vi "LVscope.vi"() -> ()   [LabVIEW 2020]
uses:
  <vilib>/Instr/_visa.llb/VISA Configure Serial Port (Instr).vi
panel:
  in  "Rising\n\nFalling":bool
  out "Triggered":bool
  out "run_ind":bool
  in  "Run/Stop":bool=TRUE
  in  "Sample rate":T1(radio)=enum."19.2 kS/s"
  in  "Trigger Voltage":dbl(knob)=2.5 scale=0.0..5.0
  out "Mean (DC)":dbl[unit]
  out "Min":dbl[unit]
  out "Max":dbl[unit]
  out "RMS":dbl[unit]
  in  "tdiv multiplier":enum32{"10us", "ms", "10ms", "100us"}(radio)=enum."ms"
  in  "Time/Div":dbl(knob)=5.0 scale=1.0..10.0
  in  "Volts/Div":sgl(knob)=2.5 caption="Diala" scale=0.1..7.5
  in  "OK Button":bool
  out "Frequency":dbl[unit]
  out "Peak to Peak":dbl[unit]
  out "Waveform Graph":waveform(dbl)(graph)
  in  "exit\nexit":bool
  in  "COM Port":refnum<visa-resource-name>
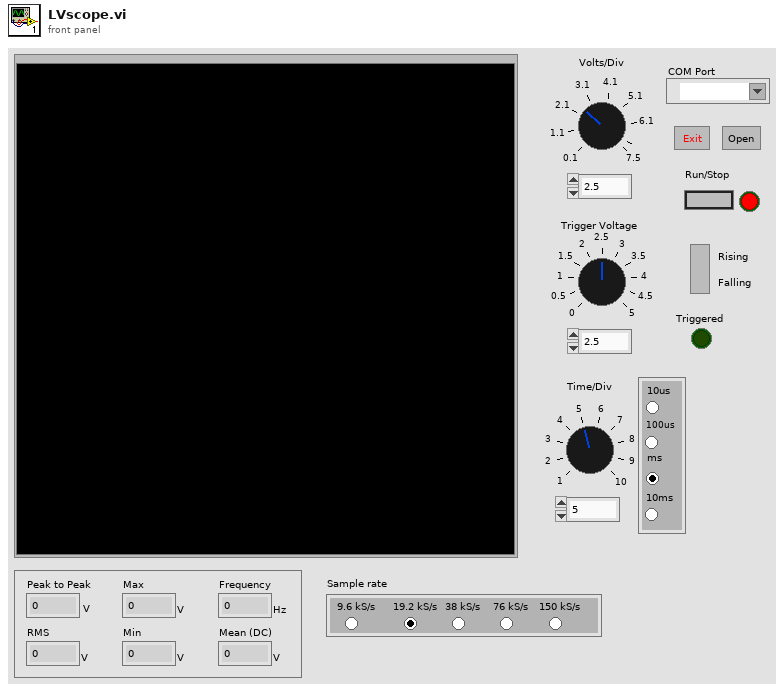
[diagram p1: front panel]
types:
  T1 = enum32{"9.6 kS/s", "19.2 kS/s", "38 kS/s", "76 kS/s", "150 kS/s"}
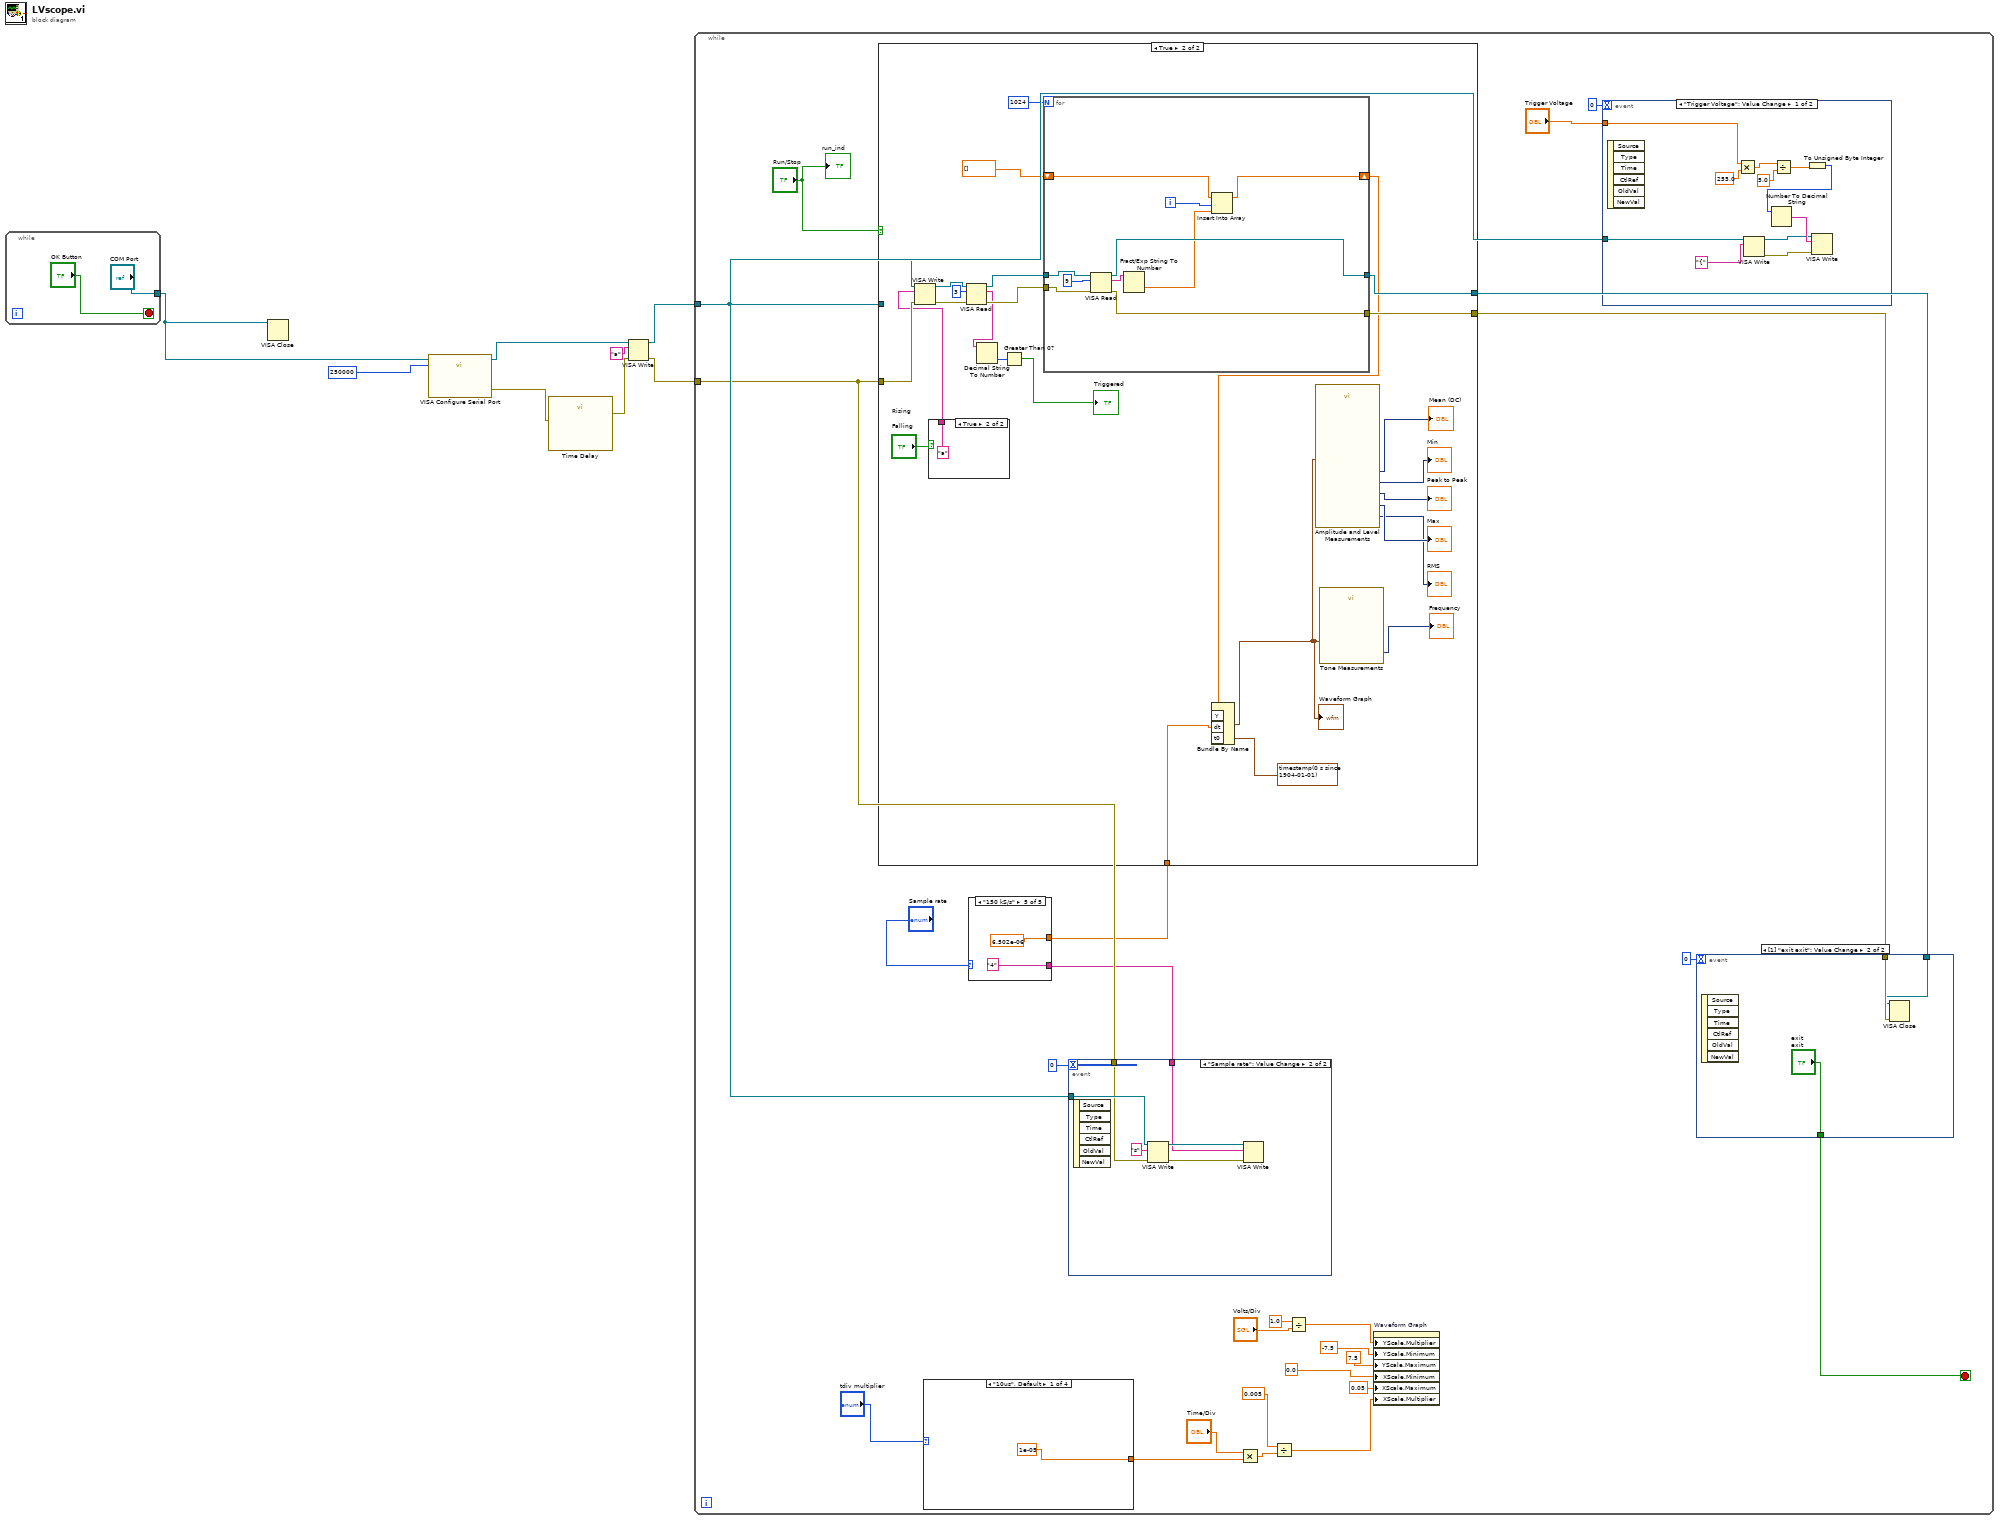
[diagram p0: block diagram]
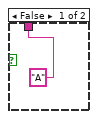
[diagram p3: hidden frame]
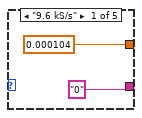
[diagram p4: hidden frame]
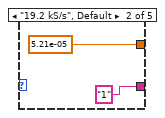
[diagram p5: hidden frame]
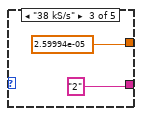
[diagram p6: hidden frame]
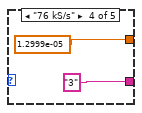
[diagram p7: hidden frame]
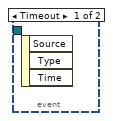
[diagram p8: hidden frame]
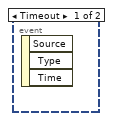
[diagram p9: hidden frame]
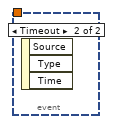
[diagram p10: hidden frame]
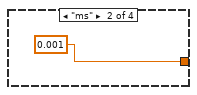
[diagram p11: hidden frame]
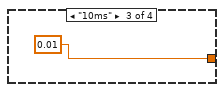
[diagram p12: hidden frame]
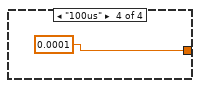
[diagram p13: hidden frame]
diagram:
  n1 = while {
    tunnel: ["COM Port"] -> w2
    stop <- "OK Button" stop-if-true
  }
  n2 = VISA Close(VISA resource name=w2) -> ()  [unwired: 1 in, 1 out]
  n3 = call-poly "VISA Configure Serial Port"("VISA resource name"=w2, "baud rate (9600)"=250000) -> ("VISA resource name out"=w6:refnum<visa-resource-name>, "error out"=w4:errorcluster)  [unwired: 12 in]
  n4 = call "Time Delay"("error in (no error)"=w4) -> ("error out"=w3:errorcluster)  [unwired: 10 in]
  n5 = VISA Write(VISA resource name=w6, write buffer="a", error in (no error)=w3) -> (VISA resource name out=w1:refnum<visa-resource-name>, error out=w5:errorcluster)  [unwired: 1 out]
  n6 = while {
    tunnel: w1 -> [w15]
    tunnel: w5 -> [w14]
    stop <- w21 stop-if-true
    n7 = case shown="\"10us\", Default" "tdiv multiplier" {
      tunnel: [1e-05 0.001 0.01 0.0001] -> w26
      frame "10us", Default {
      }
      frame "ms" {
      }
      frame "10ms" {
      }
      frame "100us" {
      }
    }
    n8 = case shown="\"150 kS/s\"" "Sample rate" {
      tunnel: ["0" "1" "2" "3" "4"] -> w13
      tunnel: [0.000104 5.21e-05 2.59994e-05 1.2999e-05 6.502e-06] -> w11
      frame "9.6 kS/s" {
      }
      frame "19.2 kS/s", Default {
      }
      frame "38 kS/s" {
      }
      frame "76 kS/s" {
      }
      frame "150 kS/s" {
      }
    }
    n9 = case shown="True" "Run/Stop" {
      tunnel: [_ w60] -> w18
      tunnel: [_ w59] -> w17
      tunnel: w15 -> [_ w58]
      tunnel: w14 -> [_ w57]
      tunnel: w11 -> [_ w53]
      frame False {
      }
      frame True {
        n10 = case shown="True" "Rising\n\nFalling" {
          tunnel: ["A" "a"] -> w37
          frame False {
          }
          frame True {
          }
        }
        n11 = VISA Write(VISA resource name=w58, write buffer=w37, error in (no error)=w57) -> (VISA resource name out=w45:refnum<visa-resource-name>, error out=w44:errorcluster)  [unwired: 1 out]
        n12 = VISA Read(VISA resource name=w45, byte count=u32 3, error in (no error)=w44) -> (VISA resource name out=w43:refnum<visa-resource-name>, read buffer=w41:string, error out=w42:errorcluster)  [unwired: 1 out]
        n13 = Decimal String To Number(string=w41) -> (number=w40:i32)  [unwired: 2 in, 1 out]
        n14 = Greater Than 0?(x=w40) -> (x > 0?=→"Triggered":bool)
        n15 = for {
          N: 1024 -> [_]
          tunnel: w43 -> [w74]
          tunnel: [w73] -> w60
          shift-right: [w67] -> w56
          shift-left: dbl[] [] ("array") -> [w68]
          tunnel: w42 -> [w66]
          tunnel: [w65] -> w59
          i -> [w70]
          n16 = VISA Read(VISA resource name=w74, byte count=u32 9, error in (no error)=w66) -> (VISA resource name out=w73:refnum<visa-resource-name>, read buffer=w71:string, error out=w65:errorcluster)  [unwired: 1 out]
          n17 = Fract/Exp String To Number(string=w71) -> (number=w69:dbl)  [unwired: 3 in, 1 out]
          n18 = Insert Into Array(array=w68, index=w70, new element=w69) -> (w67:dbl[])
        }
        n19 = Bundle By Name("Y"=w56, "dt"=w53, "t0"=timestamp(0 s since 1904-01-01)) -> (w54:waveform(dbl))  [unwired: 1 in]
        "Waveform Graph" <- w54
        n20 = call "Amplitude and Level Measurements"("Signals"=w54) -> ("Mean (DC)"=→"Mean (DC)":dynamicdata, "RMS"=→"RMS":dynamicdata, "Negative Peak"=→"Min":dynamicdata, "Positive Peak"=→"Max":dynamicdata, "Peak to Peak"=→"Peak to Peak":dynamicdata)  [unwired: 9 in, 1 out]
        n21 = call "Tone Measurements"("Signals"=w54) -> ("Frequency"=→"Frequency":dynamicdata)  [unwired: 9 in, 1 out]
      }
    }
    n22 = event shown="[1] \"Sample rate\": Value Change" {
      selector: _ -> [_ _]
      dyn-events: _ -> [_ _]
      timeout: 0 -> [_ _]
      tunnel: w15 -> [_ w87]
      tunnel: w14 -> [_ w86]
      tunnel: w13 -> [_ w85]
      event Timeout {
        n23 = event-data() -> ()  [unwired: 1 in, 3 out]
      }
      event "Sample rate": Value Change {
        n24 = event-data() -> ()  [unwired: 1 in, 6 out]
        n25 = VISA Write(VISA resource name=w87, write buffer="s", error in (no error)=w86) -> (VISA resource name out=w89:refnum<visa-resource-name>, error out=w88:errorcluster)  [unwired: 1 out]
        n26 = VISA Write(VISA resource name=w89, write buffer=w85, error in (no error)=w88) -> ()  [unwired: 3 out]
      }
    }
    n27 = Multiply(x="Time/Div", y=w26) -> (x*y=w27:dbl)
    n28 = Divide(x=0.005, y=w27) -> (x/y=w24:dbl)
    n29 = Divide(x=1.0, y="Volts/Div") -> (x/y=w34:dbl)
    n30 = property on="Waveform Graph" class="WFGraph (strict)"("YScale.Multiplier"=w34, "YScale.Minimum"=-7.5 ("Y Scale.Range:Minimum"), "YScale.Maximum"=7.5 ("Y Scale.Range:Maximum"), "XScale.Minimum"=0.0 ("X Scale.Range:Minimum"), "XScale.Maximum"=0.05 ("X Scale.Range:Maximum"), "XScale.Multiplier"=w24) -> ()  [unwired: 2 in, 2 out]
    n31 = event shown="[0] \"Trigger Voltage\": Value Change" {
      selector: _ -> [_ _]
      dyn-events: _ -> [_ _]
      timeout: 0 -> [_ _]
      tunnel: w15 -> [w95 _]
      tunnel: "Trigger Voltage" -> [w94 _]
      event "Trigger Voltage": Value Change {
        n32 = event-data() -> ()  [unwired: 1 in, 6 out]
        n33 = Multiply(x=w94, y=255.0) -> (x*y=w101:dbl)
        n34 = VISA Write(VISA resource name=w95, write buffer="{") -> (VISA resource name out=w102:refnum<visa-resource-name>, error out=w103:errorcluster)  [unwired: 1 in, 1 out]
        n35 = Divide(x=w101, y=5.0) -> (x/y=w100:dbl)
        n36 = To Unsigned Byte Integer(number=w100) -> (unsigned 8bit integer=w99:u8)
        n37 = Number To Decimal String(number=w99) -> (decimal integer string=w104:string)  [unwired: 1 in]
        n38 = VISA Write(VISA resource name=w102, write buffer=w104, error in (no error)=w103) -> ()  [unwired: 3 out]
      }
      event Timeout {
        n39 = event-data() -> ()  [unwired: 1 in, 3 out]
      }
    }
    n40 = event shown="[1] \"exit exit\": Value Change" {
      selector: _ -> [_ _]
      dyn-events: _ -> [_ _]
      timeout: 0 -> [_ _]
      tunnel: w17 -> [_ w93]
      tunnel: w18 -> [_ w92]
      tunnel: [_ "exit\nexit"] -> w21
      event Timeout {
        n41 = event-data() -> ()  [unwired: 1 in, 3 out]
      }
      event "exit\nexit": Value Change {
        n42 = event-data() -> ()  [unwired: 1 in, 6 out]
        n43 = VISA Close(VISA resource name=w92, error in (no error)=w93) -> ()  [unwired: 1 out]
      }
    }
    "run_ind" <- "Run/Stop"
  }
